vi "Calculate Initial and Final Voltages.vi"(7 "Waveform Array":waveform(dbl)[](array[waveform]), 9 "Digitizer Channel (1-4)":i32) -> (8 "Initial Voltage":dbl, 10 "Final Voltage":dbl, 15 "Peak-to-Peak Voltage":dbl)   [LabVIEW 2010]
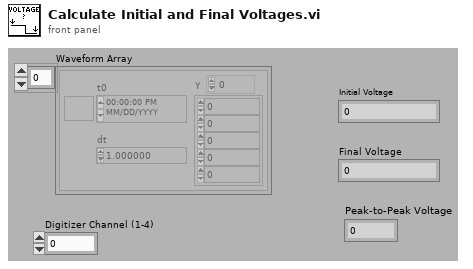
[diagram p1: front panel]
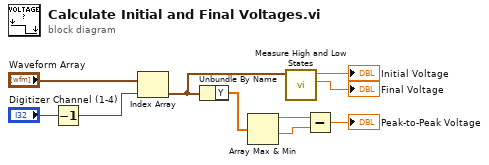
[diagram p0: block diagram]
diagram:
  n1 = Decrement(x="Digitizer Channel (1-4)") -> (x-1=w8:i32)
  n2 = Index Array(array="Waveform Array", index=w8) -> (element=w3:waveform(dbl))
  n3 = Unbundle By Name(w3) -> ("Y"=w7:dbl[])
  n4 = Array Max & Min(array=w7) -> (max value=w6:dbl, min value=w5:dbl)  [unwired: 2 out]
  n5 = call "Measure High and Low States.vi"("signal in"=w3) -> ("final state level"=→"Final Voltage":dbl, "inital state level"=→"Initial Voltage":dbl)  [unwired: 8 in, 1 out]
  n6 = Subtract(x=w6, y=w5) -> (x-y=→"Peak-to-Peak Voltage":dbl)
